vi "Cost.vi"(8 "error in (no error)":errorcluster caption="错误输入（无错误）", 11 "House Blend Coffee 输入":refnum<class "House Blend Coffee.lvclass">) -> (0 "error out":errorcluster caption="错误输出", 2 "cost":dbl, 3 "House Blend Coffee 输出":refnum<class "House Blend Coffee.lvclass">)   [LabVIEW 2016, in "House Blend Coffee.lvclass"]
uses:
  House Blend Coffee.lvclass
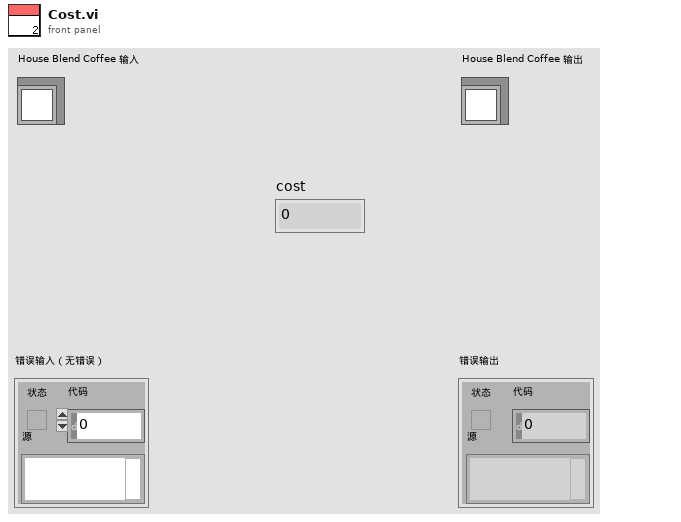
[diagram p1: front panel]
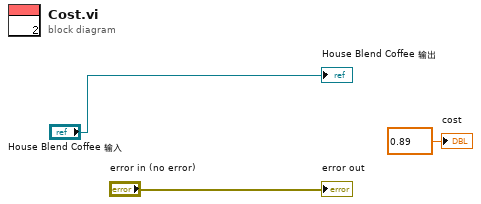
[diagram p0: block diagram]
diagram:
  "error out" <- "error in (no error)"
  "House Blend Coffee 输出" <- "House Blend Coffee 输入"
  "cost" <- 0.89 ("cost")
